vi "Init Events.vi"(8 "error in (no error)":errorcluster, 11 "AsyncClassTemplate in":refnum<class "AsyncClassTemplate.lvclass">) -> (0 "error out":errorcluster, 3 "AsyncClassTemplate out":refnum<class "AsyncClassTemplate.lvclass">)   [LabVIEW 2020, in "Vecto.lvlib" / "AsyncClassTemplate.lvclass"]
uses:
  AsyncClassTemplate.lvclass
  Incoming Events.ctl
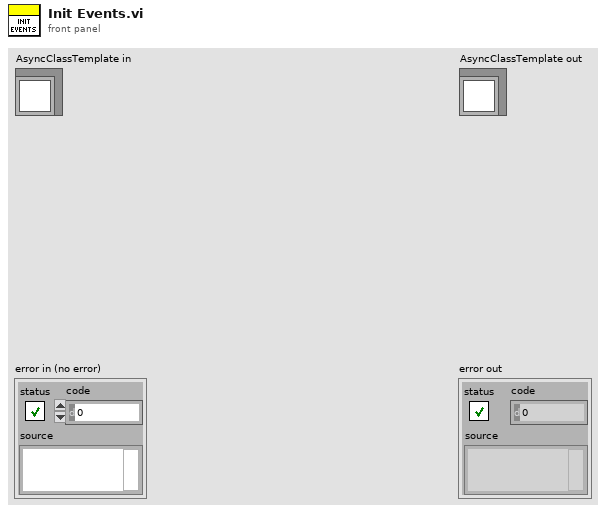
[diagram p1: front panel]
types:
  T1 = typedef "Vecto.lvlib/AsyncClassTemplate.lvclass/Incoming Events.ctl" = cluster{"Close":refnum<user-event>}
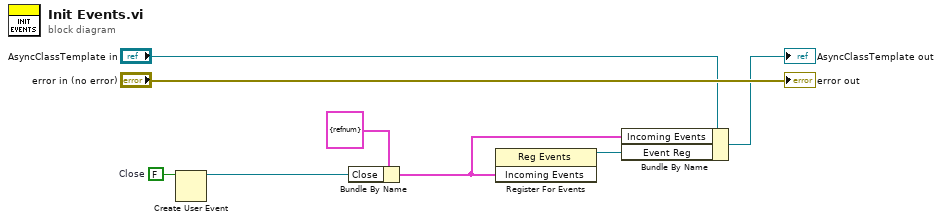
[diagram p0: block diagram]
diagram:
  w7 = FALSE  # Close
  n1 = Create User Event(user event datatype=w7) -> (user event=w5:refnum<user-event>)  [unwired: 1 in, 1 out]
  n2 = Bundle By Name(cluster=T1 {"Close"=refnum} ("Incoming Events"), "Close"=w5) -> (w3:T1)
  n3 = register-events(w3) -> (reference out=w4:refnum<event-registration>)  [unwired: 2 in, 1 out]
  n4 = Bundle By Name(cluster="AsyncClassTemplate in", "Incoming Events"=w3, "Event Reg"=w4) -> (→"AsyncClassTemplate out":refnum<class "AsyncClassTemplate.lvclass">)
  "error out" <- "error in (no error)"
